vi "Encoder Math Steering.vi"(0 "Encoder B":bool, 5 "Encoder A":bool, 13 "Encoder Index":bool) -> (3 "Count Delta":i32, 4 "The Encoder Changed":bool, 6 "Count Zeroed at Index":i32, 14 "Current count":i32)   [LabVIEW 2009]
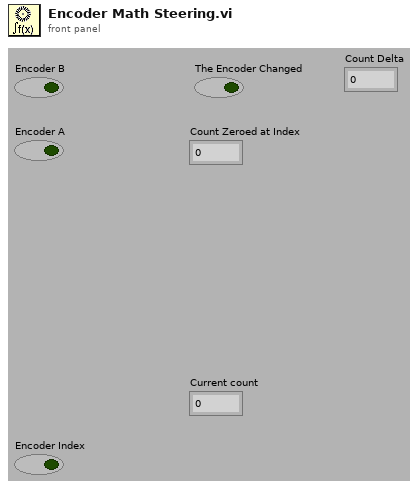
[diagram p1: front panel]
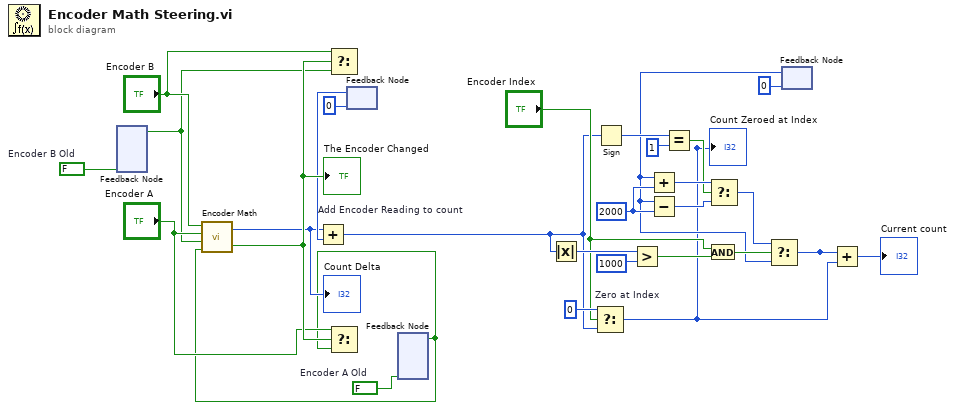
[diagram p0: block diagram]
diagram:
  w2 = FALSE  # Encoder A Old
  w5 = FALSE  # Encoder B Old
  w26 = 2000 ("y")
  n1 = feedback #1(w5) -> (w4:bool)
  n2 = feedback #2(0) -> (w14:i32)
  n3 = feedback #3(w2) -> (w1:bool)
  n4 = call "Encoder Math.vi"("Encoder A_old"=w1, "Encoder B_old"=w4, "Encoder A_new"="Encoder A", "Encoder B_new"="Encoder B") -> ("The Encoder Changed"=w29:bool, "Change in Encoder Value"=w6:i32)
  "The Encoder Changed" <- w29
  "Count Delta" <- w6
  n5 = Add "Add Encoder Reading to count"(x=w6, y=w14) -> (x+y=w7:i32)
  n6 = Select(t="Encoder B", s=w29, f=w4) -> (s? t:f=w30:bool)
  n7 = Select(t="Encoder A", s=w29, f=w1) -> (s? t:f=w3:bool)
  n8 = Absolute Value(x=w7) -> (abs(x)=w19:i32)
  n9 = Select "Zero at Index"(t=0 ("Zero at Index"), s="Encoder Index", f=w7) -> (s? t:f=w9:i32)
  "Count Zeroed at Index" <- w9
  n10 = Sign(1:w7) -> (0:w23:i32)
  n11 = Greater?(x=w19, y=1000) -> (0:w17:bool)
  n12 = Equal?(x=w23, y=1) -> (x = y?=w22:bool)
  n13 = And(x="Encoder Index", y=w17) -> (x .and. y?=w15:bool)
  n14 = feedback #4(0) -> (w12:i32)
  n15 = Add(x=w12, y=w26) -> (x+y=w25:i32)
  n16 = Subtract(x=w12, y=w26) -> (x-y=w24:i32)
  n17 = Select(t=w25, s=w22, f=w24) -> (s? t:f=w20:i32)
  n18 = Select(t=w20, s=w15, f=w12) -> (s? t:f=w10:i32)
  n19 = Add(x=w10, y=w9) -> (x+y=→"Current count":i32)
